vi "ROI Min Max.vi"(10 "ROI 2":dbl, 11 "ROI 1":dbl) -> (2 "ROI Max":dbl, 3 "ROI Min":dbl)   [LabVIEW 2023]
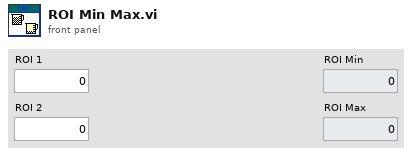
[diagram p1: front panel]
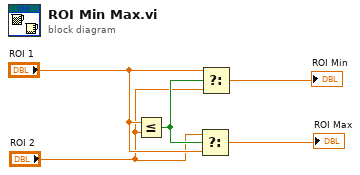
[diagram p0: block diagram]
diagram:
  n1 = Less Or Equal?(x="ROI 1", y="ROI 2") -> (x <= y?=w5:bool)
  n2 = Select(t="ROI 2", s=w5, f="ROI 1") -> (s? t:f=→"ROI Max":dbl)
  n3 = Select(t="ROI 1", s=w5, f="ROI 2") -> (s? t:f=→"ROI Min":dbl)
